vi "SEE_PXI_TopBench_Rev11.vi"() -> ()   [LabVIEW 2019]
uses:
  Controls/DataBlockControl.ctl
  Controls/RFBlockControl.ctl
  <instrlib>/niScope/Controls/niScope vertical coupling.ctl
  Controls/PlotColorArray.ctl
panel:
  out "OscilloscopeInfoArray":T2(array[cluster]) {"vertical coupling" items=["AC", "DC", "Ground"]}
  out "DCPowerInfoArray":T3(array[cluster])
  out "RFBlockInfoArray":T4[](array[typedef])
  out "error in":errorcluster
  out "VISAPowerInfoArray":T5(array[cluster])
  out "Run Parameters":T6
  in  "stop":bool
  out "Configuration Dashboard":bool[](array[boolean])
  in  "Data Collection Block":bool
  in  "Oscilloscope Block":bool
  in  "Power Block":bool
  in  "RF Block":bool
  in  "Data Block":bool
  in  "Reset":bool
  # "Instructions:\nProgress through the configuration dashboard, note the arrays to the right to confirm settings. Once everything is configured, you can begin data collection"
  # "IMPORTANT NOTES\n\nALL LEDs must be lit up before you can begin data collection. Even if you don't need an RF source or oscilloscope, you still just open up the system and then exit (you don't need to configure one.\n\nAfter data collection, you will have the option to reset the system or keep the configuration.\n\nOnly press \"stop\" if you are completely done with collecting data or if the program does not allow you to open another subvi\n\nIf you get a \"running an implicit call\" just restart the program"
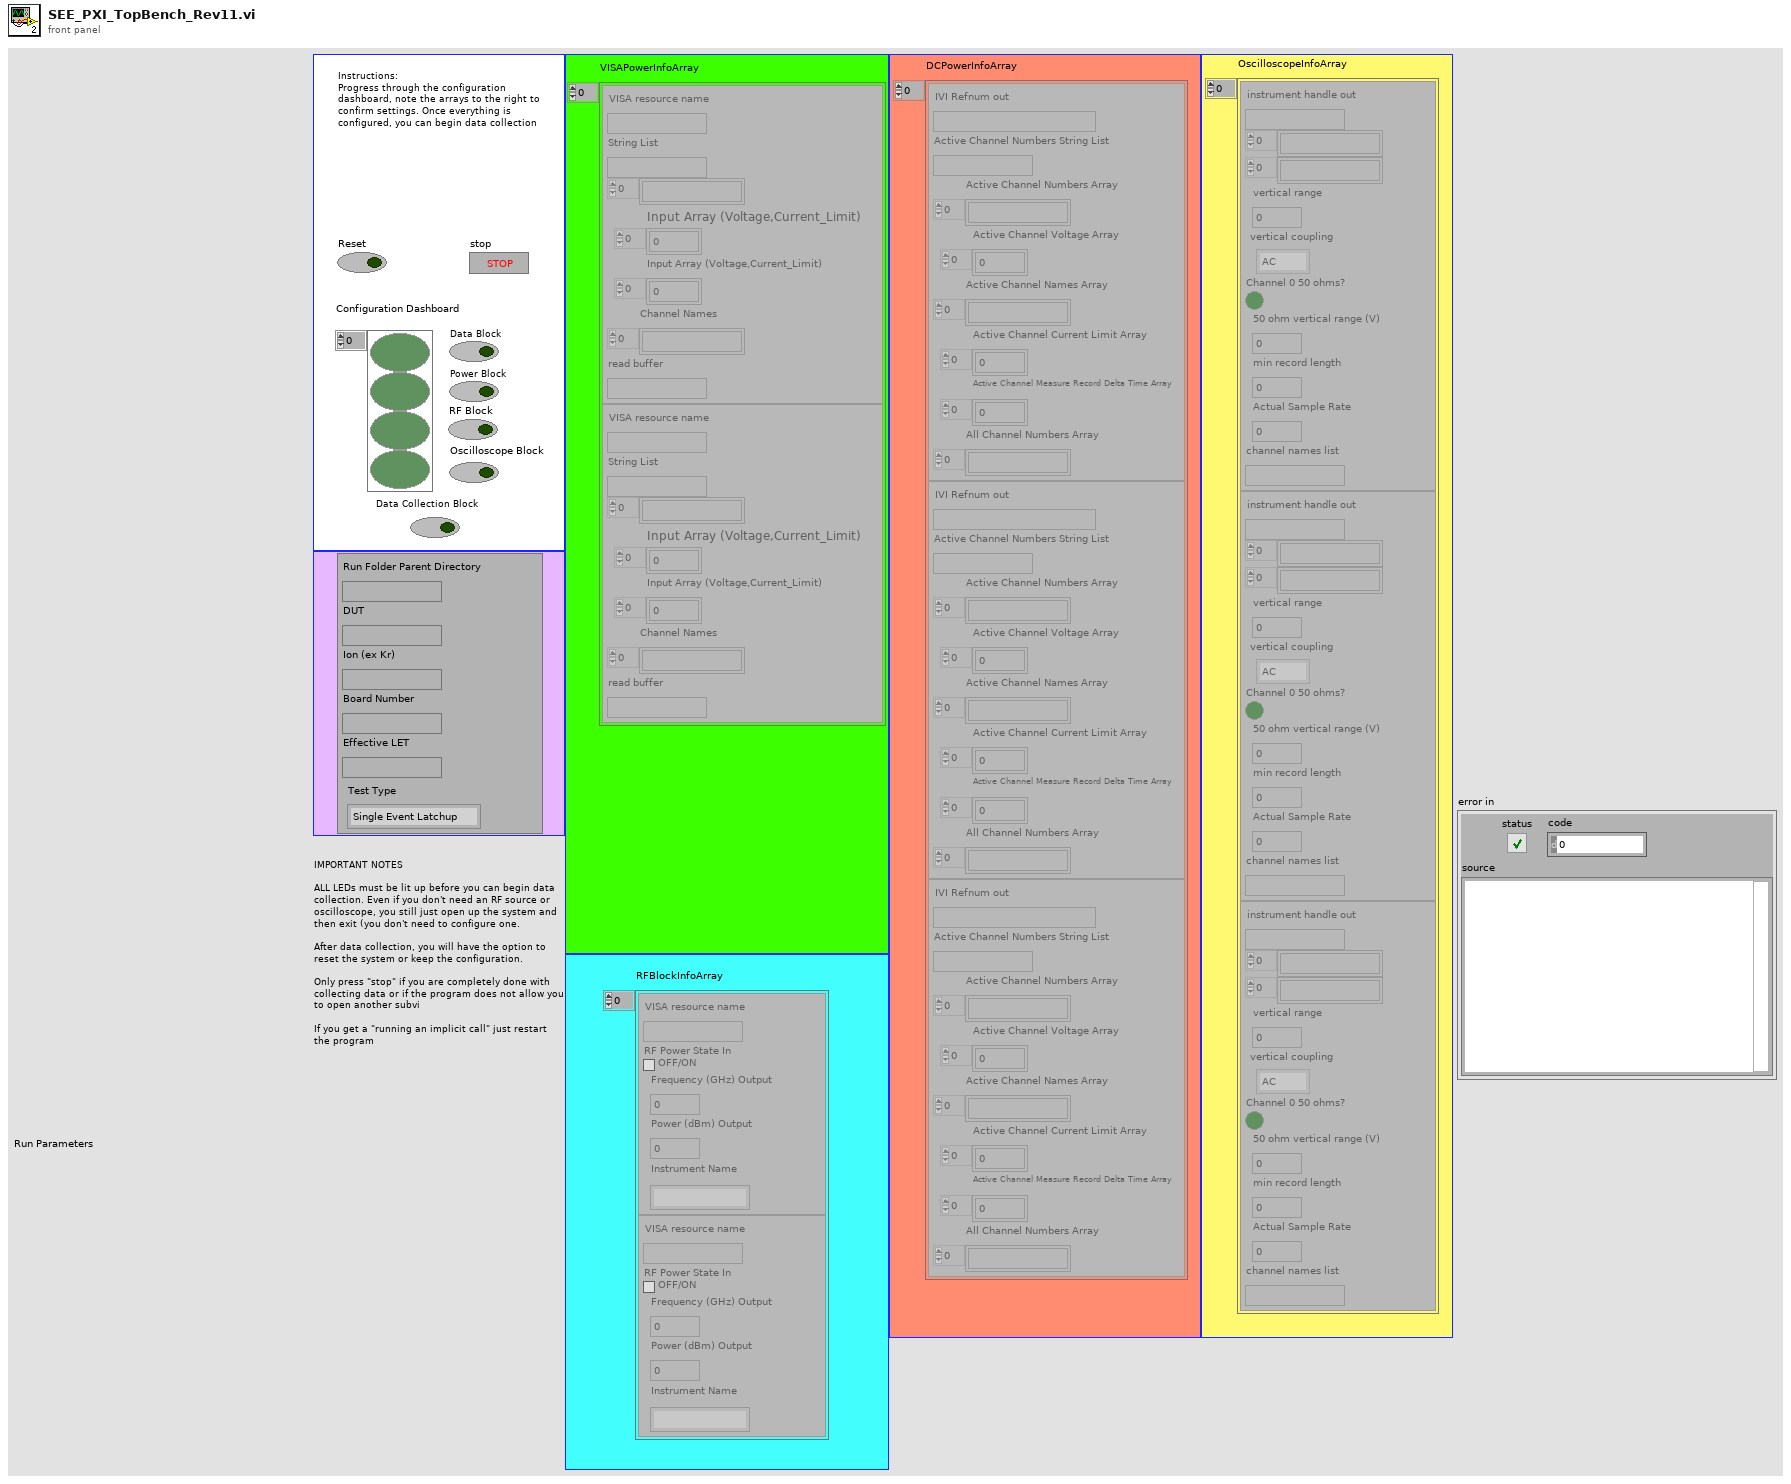
[diagram p1: front panel]
types:
  T1 = typedef "niScope vertical coupling.ctl" = i32
  T2 = cluster{"instrument handle out":refnum<k15>, string[], string[], "vertical range":dbl, "vertical coupling":T1, "Channel 0 50 ohms?":bool, "50 ohm vertical range (V)":dbl, "min record length":i32, "Actual Sample Rate":dbl, "channel names list":string}[]
  T3 = cluster{"IVI Refnum out":refnum<k15>, "Active Channel Numbers String List":string, "Active Channel Numbers Array":string[], "Active Channel Voltage Array":dbl[], "Active Channel Names Array":string[], "Active Channel Current Limit Array":dbl[], "Active Channel Measure Record Delta Time Array":dbl[], "All Channel Numbers Array":string[]}[]
  T4 = typedef "RFBlockControl.ctl" = cluster{"VISA resource name":refnum<visa-resource-name>, "RF Power State In":bool, "Frequency (GHz) Output":dbl, "Power (dBm) Output":dbl, "Instrument Name":string}
  T5 = cluster{"VISA resource name":refnum<visa-resource-name>, "String List":string, string[], "Input Array (Voltage,Current_Limit)":dbl[], "Input Array (Voltage,Current_Limit)":dbl[], "Channel Names":string[], "read buffer":string}[]
  T6 = typedef "DataBlockControl.ctl" = cluster{"Run Folder Parent Directory":path, "DUT":string, "Ion (ex Kr)":string, "Board Number":string, "Effective LET":string, "Test Type":enum16{"Single Event Latchup", "Single Event Transient", "Single Event Upset"}}
  T7 = typedef "PlotColorArray.ctl" = u32[]
  T8 = cluster{"instrument handle out":refnum<k15>, string, string[], dbl[], string[], "Current Limit Output Array":dbl[], dbl[]}[]
  T9 = cluster{"instrument handle out":refnum<k15>, "channel numbers array":string[], "channel names array":string[], "vertical range":dbl, "vertical coupling":T1, "Channel 0 50 ohms?":bool, "50 ohm vertical range (V)":dbl, "min record length":i32, "Actual Sample Rate":dbl}[]
  T10 = cluster{"Array of fetched data":dbl[][], string, i32[]}[]
  T11 = cluster{"Array of fetched data":dbl[][], string, i32[]}[][]
  T12 = cluster{"Array of fetched data":dbl[][], string, i32[]}
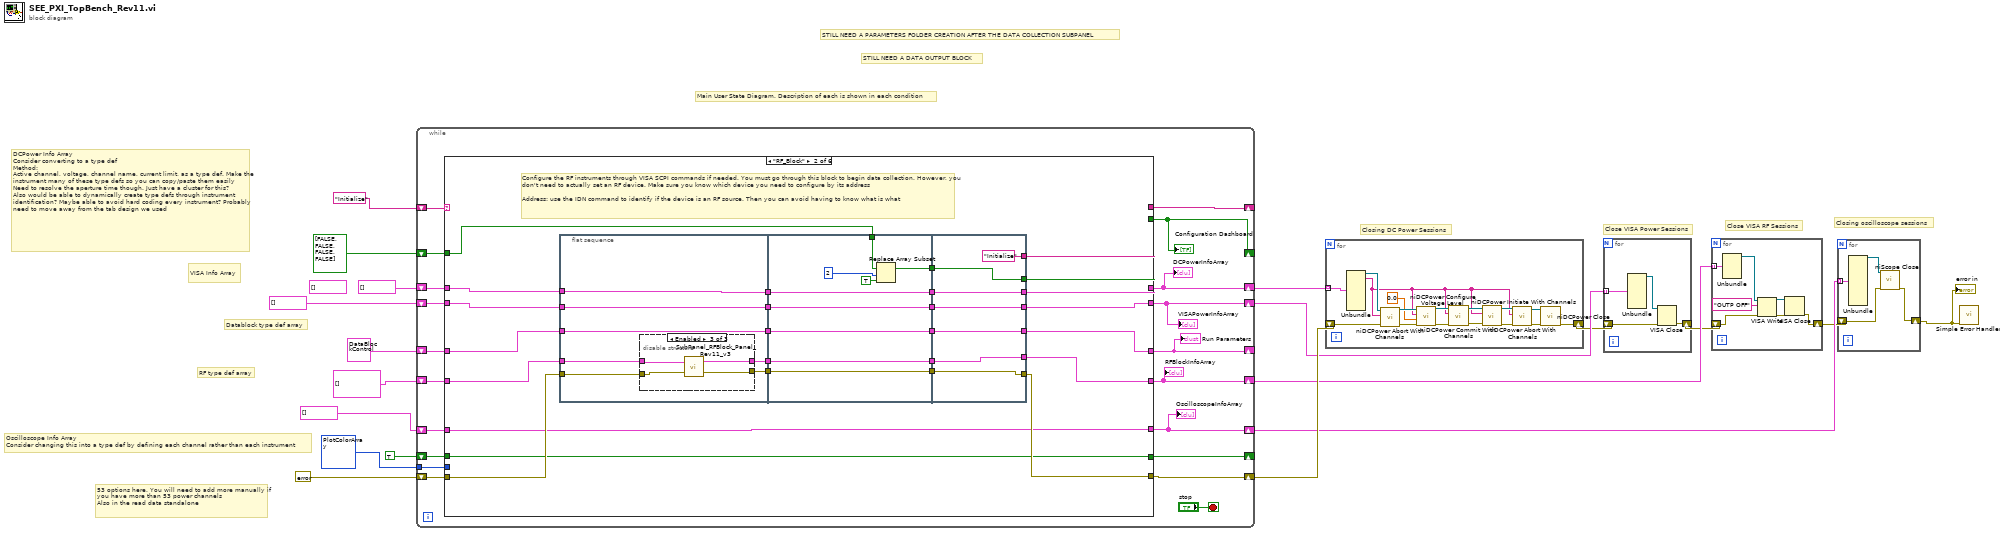
[diagram p0: block diagram]
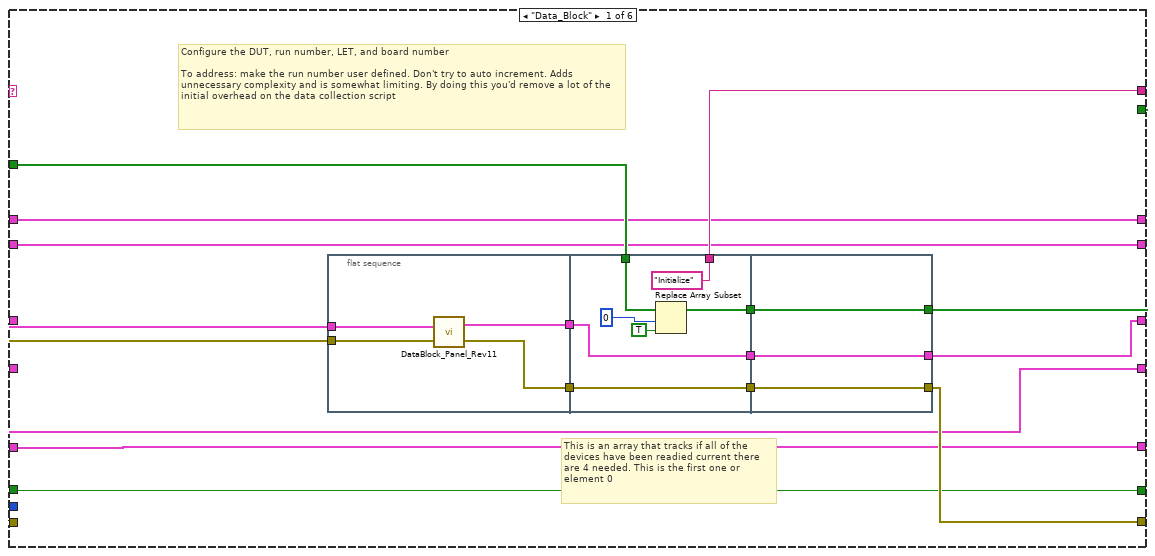
[diagram p2: hidden frame]
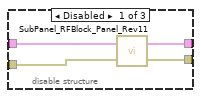
[diagram p3: hidden frame]
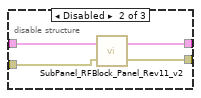
[diagram p4: hidden frame]
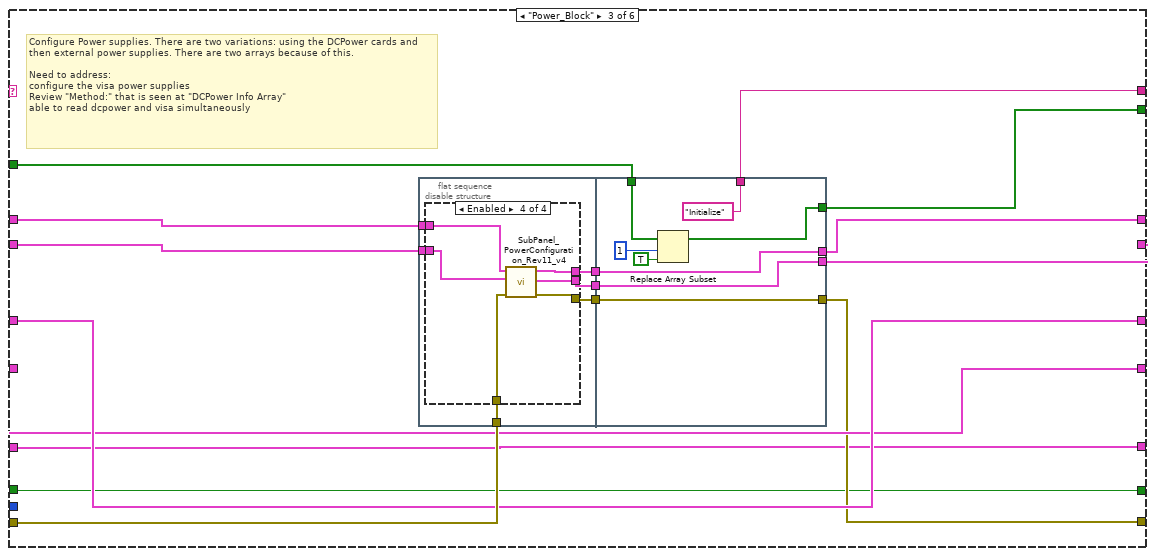
[diagram p5: hidden frame]
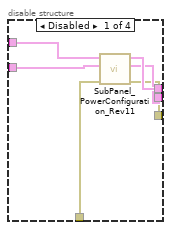
[diagram p6: hidden frame]
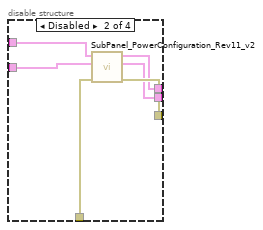
[diagram p7: hidden frame]
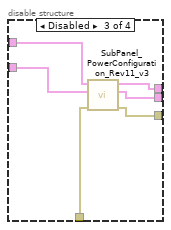
[diagram p8: hidden frame]
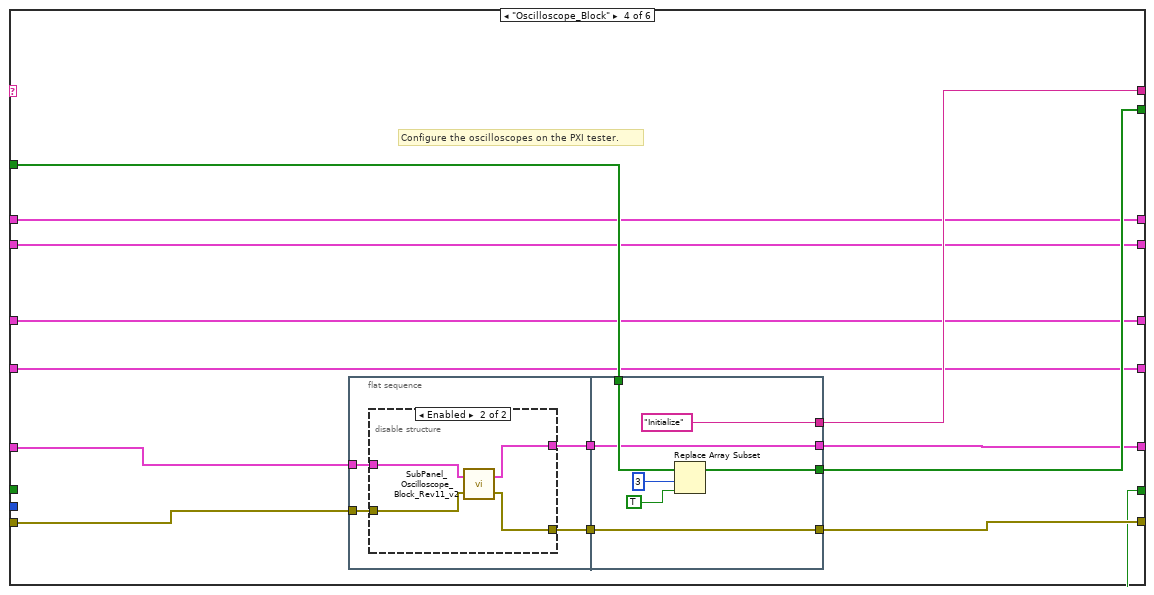
[diagram p9: hidden frame]
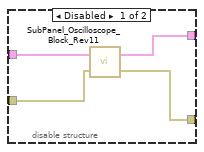
[diagram p10: hidden frame]
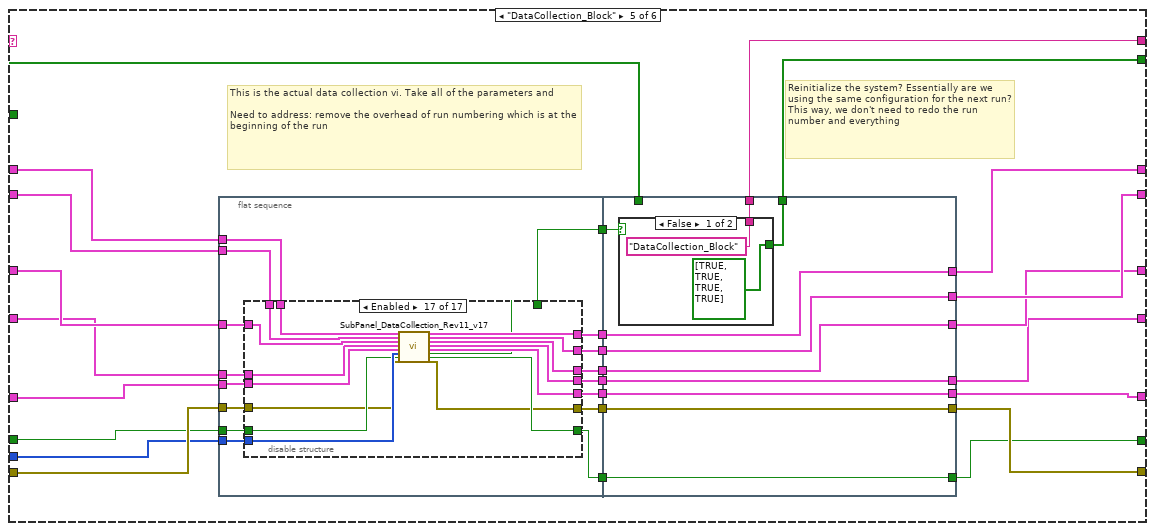
[diagram p11: hidden frame]
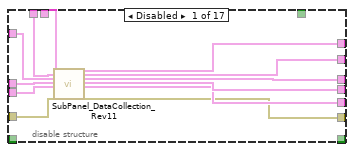
[diagram p12: hidden frame]
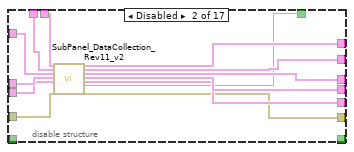
[diagram p13: hidden frame]
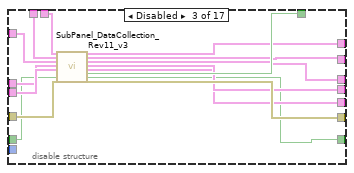
[diagram p14: hidden frame]
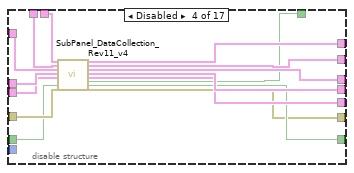
[diagram p15: hidden frame]
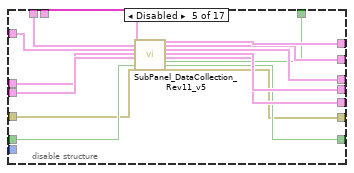
[diagram p16: hidden frame]
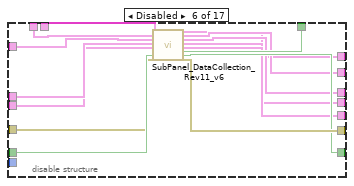
[diagram p17: hidden frame]
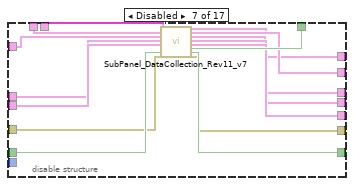
[diagram p18: hidden frame]
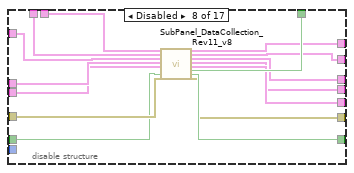
[diagram p19: hidden frame]
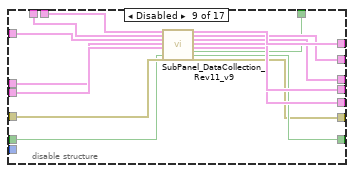
[diagram p20: hidden frame]
diagram:
  (unwired) T8 [] ("DCPowerInformationClusterArray_Input")
  # "Closing oscilloscope sessions"
  # "DCPower Info Array\nConsider converting to a type def\nMethod:\nActive channel, voltage, channel name, current limit, as a type def. Make the instrument many of these type defs so you can copy/paste them easily\nNeed to resolve the aperture time though. Just have a cluster for this?\nAlso would be able to dynamically create type defs through instrument identification? Maybe able to avoid hard coding every instrument? Probably need to move away from the tab design we used"
  # "Datablock type def array"
  # "RF type def array"
  # "Main User State Diagram. Description of each is shown in each condition"
  # "53 options here. You will need to add more manually if you have more than 53 power channels\nAlso in the read data standalone"
  # "STILL NEED A DATA OUTPUT BLOCK"
  # "STILL NEED A PARAMETERS FOLDER CREATION AFTER THE DATA COLLECTION SUBPANEL"
  # "Close VISA RF Sessions"
  # "Close VISA Power Sessions"
  # "Closing DC Power Sessions"
  # "Oscilloscope Info Array\nConsider changing this into a type def by defining each channel rather than each instrument"
  # "VISA Info Array"
  n1 = while {
    shift-right: [w37] -> _
    shift-left: bool[] [FALSE, FALSE, FALSE, FALSE] -> [w38]
    shift-right: [w36] -> _
    shift-left: "Initialize" -> [w39]
    shift-right: [w33] -> w13
    shift-left: errorcluster {"status"=FALSE, "code"=0, "source"=""} ("error in") -> [w34]
    shift-right: [w31] -> _
    shift-left: T6 {"Run Folder Parent Directory"=path "", "DUT"="", "Ion (ex Kr)"="", "Board Number"="", "Effective LET"="", "Test Type"=enum."Single Event Latchup"} ("Run Data SubPanel Input") -> [w32]
    shift-right: [w29] -> w10
    shift-left: T4[] [] ("RF Block Input Array") -> [w30]
    shift-right: [w25] -> w14
    shift-left: T3 [] ("DCPowerInformationClusterArray_Input") -> [w28]
    shift-right: [w26] -> w12
    shift-left: T5 [] ("VISAPowerInfoInputArray") -> [w27]
    shift-right: [w23] -> w6
    shift-left: T2 [] ("Oscilloscope Configuration Input Array") -> [w24]
    shift-right: [w21] -> _
    shift-left: TRUE ("New Run?") -> [w22]
    tunnel: T7 [16711686, 65351, 8978420, 14474240, 16139007, 16752640, 8958719, 16758973, 16777215, 46792, 11992992, 12961221, 16763690, 12600063, 16711835, 2953983, 40796, 13111296, 13352613, 9221011, 12964076, 12819897, 65442, 16776704, 14540253, 16740729, 10658047, 10813344, 16753521, 13413843, 8691115, 10339240, 14401205, 16746704, 7467519, 16775978, 13872558, 11387603, 13354405, 10420227, 13107364, 4060, 35208, 11817216, 7566080, 40796, 7539456, 2837073, 6372186, 7499083, 10648702, 16757152] ("Array") -> [w20]
    stop <- "stop" stop-if-true
    n2 = case shown="\"RF_Block\"" w39 {
      selector: w39 -> [_ _ _ _ _ w551]
      tunnel: w38 -> [w56 w93 w142 w199 w227 w553]
      tunnel: [w55 w92 w141 w198 w226 w552] -> w37
      tunnel: [w53 w96 w140 w197 w225 w549] -> w36
      tunnel: w34 -> [w52 w95 w145 w192 w239 w547]
      tunnel: [w51 w94 w134 w191 w229 w547] -> w33
      tunnel: w32 -> [w48 w82 w144 w194 w242 w546]
      tunnel: [w47 w81 w144 w194 w234 w546] -> w31
      tunnel: w30 -> [w44 w88 w143 w193 w241 w545]
      tunnel: [w44 w87 w143 w193 w232 w545] -> w29
      tunnel: w28 -> [w43 w77 w147 w196 w244 w544]
      tunnel: w27 -> [w42 w73 w146 w195 w243 w543]
      tunnel: [w43 w80 w139 w196 w238 w544] -> w25
      tunnel: [w42 w76 w137 w195 w236 w543] -> w26
      tunnel: w24 -> [w41 w72 w133 w189 w240 w542]
      tunnel: [w41 w72 w133 w188 w219 w542] -> w23
      tunnel: w22 -> [w40 w71 w132 w186 w223 w541]
      tunnel: [w40 w71 w132 w186 w221 w541] -> w21
      tunnel: w20 -> [_ _ _ _ w220 _]
      frame "Data_Block" {
        # "This is an array that tracks if all of the devices have been readied current there are 4 needed. This is the first one or element 0"
        # "Configure the DUT, run number, LET, and board number\n\nTo address: make the run number user defined. Don't try to auto increment. Adds unnecessary complexity and is somewhat limiting. By doing this you'd remove a lot of the initial overhead on the data collection script"
        n3 = flat-sequence {
          tunnel: w52 -> [w60]
          tunnel: [w59] -> w49
          tunnel: w48 -> [w58]
          tunnel: [w57] -> w45
          tunnel: w56 -> [w67]
          tunnel: [w64] -> w54
          tunnel: ["Initialize"] -> w53
          tunnel: [w62] -> w50
          tunnel: w49 -> [w62]
          tunnel: [w61] -> w46
          tunnel: w45 -> [w61]
          tunnel: [w70] -> w55
          tunnel: w54 -> [w70]
          tunnel: [w69] -> w51
          tunnel: w50 -> [w69]
          tunnel: [w68] -> w47
          tunnel: w46 -> [w68]
          frame #0 {
            n4 = call "DataBlock_Panel_Rev11.vi"("error in"=w60, "Run Data SubPanel Input"=w58) -> ("error out"=w59:errorcluster, "Run Data SubPanel Output"=w57:T6)
          }
          frame #1 {
            n5 = Replace Array Subset(array=w67, new element=TRUE ("new element/subarray"), index=0) -> (w64:bool[])
          }
          frame #2 {
          }
        }
      }
      frame "RF_Block" {
        # "Configure the RF instruments through VISA SCPI commands if needed. You must go through this block to begin data collection. However, you don't need to actually set an RF device. Make sure you know which device you need to configure by its address\n\nAddress: use the IDN command to identify if the device is an RF source. Then you can avoid having to know what is what"
        n6 = flat-sequence {
          tunnel: w95 -> [w103]
          tunnel: [w102] -> w89
          tunnel: w88 -> [w101]
          tunnel: [w100] -> w85
          tunnel: [w99] -> w83
          tunnel: w82 -> [w99]
          tunnel: [w98] -> w78
          tunnel: w77 -> [w98]
          tunnel: [w97] -> w74
          tunnel: w73 -> [w97]
          tunnel: w93 -> [w124]
          tunnel: [w121] -> w91
          tunnel: [w120] -> w90
          tunnel: w89 -> [w120]
          tunnel: [w119] -> w86
          tunnel: w85 -> [w119]
          tunnel: [w118] -> w84
          tunnel: w83 -> [w118]
          tunnel: [w117] -> w79
          tunnel: w78 -> [w117]
          tunnel: [w116] -> w75
          tunnel: w74 -> [w116]
          tunnel: ["Initialize"] -> w96
          tunnel: [w129] -> w94
          tunnel: [w130] -> w92
          tunnel: w91 -> [w130]
          tunnel: w90 -> [w129]
          tunnel: [w128] -> w87
          tunnel: w86 -> [w128]
          tunnel: [w127] -> w81
          tunnel: w84 -> [w127]
          tunnel: [w126] -> w80
          tunnel: w79 -> [w126]
          tunnel: [w125] -> w76
          tunnel: w75 -> [w125]
          frame #0 {
            n7 = disable-structure shown="Enabled" {
              disable-tunnel: w103 -> [w107 w110 w114]
              disable-tunnel: [w106 w108 w113] -> w102
              disable-tunnel: w101 -> [w105 w111 w115]
              disable-tunnel: [w104 w109 w112] -> w100
              frame Disabled {
                n8 = call "SubPanel_RFBlock_Panel_Rev11.vi"("error input"=w107, "RF Block Input"=w105) -> ("error output"=w106:errorcluster, "RF Block Output"=w104:T4)
              }
              frame Disabled {
                n9 = call "SubPanel_RFBlock_Panel_Rev11_v2.vi"("error input"=w110, "RF Block Input Array"=w111) -> ("error output"=w108:errorcluster, "RF Block Output Array"=w109:T4[])
              }
              frame Enabled {
                n10 = call "SubPanel_RFBlock_Panel_Rev11_v3.vi"("error input"=w114, "RF Block Input Array"=w115) -> ("error output"=w113:errorcluster, "RF Block Output Array"=w112:T4[])
              }
            }
          }
          frame #1 {
            n11 = Replace Array Subset(array=w124, new element=TRUE ("new element/subarray"), index=2) -> (w121:bool[])
          }
          frame #2 {
          }
        }
      }
      frame "Power_Block" {
        # "Configure Power supplies. There are two variations: using the DCPower cards and then external power supplies. There are two arrays because of this.  \n\nNeed to address:\nconfigure the visa power supplies\nReview \"Method:\" that is seen at \"DCPower Info Array\"\nable to read dcpower and visa simultaneously"
        n12 = flat-sequence {
          tunnel: w147 -> [w153]
          tunnel: w146 -> [w152]
          tunnel: w145 -> [w151]
          tunnel: [w150] -> w138
          tunnel: [w149] -> w136
          tunnel: [w148] -> w135
          tunnel: w142 -> [w183]
          tunnel: [w182] -> w141
          tunnel: ["Initialize"] -> w140
          tunnel: [w180] -> w139
          tunnel: w138 -> [w180]
          tunnel: [w179] -> w137
          tunnel: w136 -> [w179]
          tunnel: [w178] -> w134
          tunnel: w135 -> [w178]
          frame #0 {
            n13 = disable-structure shown="Enabled" {
              disable-tunnel: w153 -> [w159 w160 w168 w173]
              disable-tunnel: w152 -> [w158 w161 w167 w172]
              disable-tunnel: w151 -> [w157 w165 w166 w177]
              disable-tunnel: [w156 w162 w169 w174] -> w150
              disable-tunnel: [w155 w163 w170 w175] -> w149
              disable-tunnel: [w154 w164 w171 w176] -> w148
              frame Disabled {
                n14 = call "SubPanel_PowerConfiguration_Rev11.vi"("error in"=w157, "VISAPowerInfoInputArray"=w158, "DCPowerInformationClusterArray_Input"=w159) -> ("error out"=w154:errorcluster, "VISAPowerInfoOutputArray"=w155:T5, "DCPowerInformationClusterArray_Output"=w156:T8)  [unwired: 6 in]
              }
              frame Disabled {
                n15 = call "SubPanel_PowerConfiguration_Rev11_v2.vi"("error in"=w165, "VISAPowerInfoInputArray"=w161, "DCPowerInformationClusterArray_Input"=w160) -> ("error out"=w164:errorcluster, "VISAPowerInfoOutputArray"=w163:T5, "DCPowerInformationClusterArray_Output"=w162:T3)  [unwired: 6 in]
              }
              frame Disabled {
                n16 = call "SubPanel_PowerConfiguration_Rev11_v3.vi"("error in"=w166, "VISAPowerInfoInputArray"=w167, "DCPowerInformationClusterArray_Input"=w168) -> ("error out"=w171:errorcluster, "VISAPowerInfoOutputArray"=w170:T5, "DCPowerInformationClusterArray_Output"=w169:T3)  [unwired: 6 in]
              }
              frame Enabled {
                n17 = call "SubPanel_PowerConfiguration_Rev11_v4.vi"("error in"=w177, "VISAPowerInfoInputArray"=w172, "DCPowerInformationClusterArray_Input"=w173) -> ("error out"=w176:errorcluster, "VISAPowerInfoOutputArray"=w175:T5, "DCPowerInformationClusterArray_Output"=w174:T3)  [unwired: 6 in]
              }
            }
          }
          frame #1 {
            n18 = Replace Array Subset(array=w183, new element=TRUE ("new element/subarray"), index=1) -> (w182:bool[])
          }
        }
      }
      frame "Oscilloscope_Block" {
        # "Configure the oscilloscopes on the PXI tester."
        n19 = flat-sequence {
          tunnel: w192 -> [w203]
          tunnel: [w202] -> w190
          tunnel: w189 -> [w201]
          tunnel: [w200] -> w187
          tunnel: w199 -> [w218]
          tunnel: [w215] -> w198
          tunnel: ["Initialize"] -> w197
          tunnel: [w213] -> w191
          tunnel: w190 -> [w213]
          tunnel: [w212] -> w188
          tunnel: w187 -> [w212]
          frame #0 {
            n20 = disable-structure shown="Enabled" {
              disable-tunnel: w203 -> [w207 w209]
              disable-tunnel: [w206 w208] -> w202
              disable-tunnel: w201 -> [w205 w211]
              disable-tunnel: [w204 w210] -> w200
              frame Disabled {
                n21 = call "SubPanel_Oscilloscope_Block_Rev11.vi"("error input"=w207, "Oscilloscope Configuration Input Array"=w205) -> ("error out"=w206:errorcluster, "Oscilloscope Configuration Output Array"=w204:T9)
              }
              frame Enabled {
                n22 = call "SubPanel_Oscilloscope_Block_Rev11_v2.vi"("error input"=w209, "Oscilloscope Configuration Input Array"=w211) -> ("error out"=w208:errorcluster, "Oscilloscope Configuration Output Array"=w210:T2)
              }
            }
          }
          frame #1 {
            n23 = Replace Array Subset(array=w218, new element=TRUE ("new element/subarray"), index=3) -> (w215:bool[])
          }
        }
      }
      frame "DataCollection_Block" {
        # "Reinitialize the system? Essentially are we using the same configuration for the next run? This way, we don't need to redo the run number and everything"
        # "This is the actual data collection vi. Take all of the parameters and \n\nNeed to address: remove the overhead of run numbering which is at the beginning of the run"
        n24 = flat-sequence {
          tunnel: w244 -> [w260]
          tunnel: w243 -> [w259]
          tunnel: w242 -> [w258]
          tunnel: w241 -> [w257]
          tunnel: w240 -> [w256]
          tunnel: w239 -> [w255]
          tunnel: [w254] -> w237
          tunnel: [w253] -> w235
          tunnel: [w252] -> w233
          tunnel: [w251] -> w231
          tunnel: [w250] -> w230
          tunnel: [w249] -> w228
          tunnel: [w248] -> w224
          tunnel: w223 -> [w247]
          tunnel: [w246] -> w222
          tunnel: w220 -> [w245]
          tunnel: [w534] -> w238
          tunnel: w237 -> [w534]
          tunnel: [w533] -> w236
          tunnel: w235 -> [w533]
          tunnel: [w532] -> w234
          tunnel: w233 -> [w532]
          tunnel: [w531] -> w232
          tunnel: w231 -> [w531]
          tunnel: [w530] -> w219
          tunnel: w230 -> [w530]
          tunnel: [w529] -> w229
          tunnel: w228 -> [w529]
          tunnel: w227 -> [_]
          tunnel: [w528] -> w226
          tunnel: [w527] -> w225
          tunnel: w224 -> [w526]
          tunnel: [w525] -> w221
          tunnel: w222 -> [w525]
          frame #0 {
            n25 = disable-structure shown="Enabled" {
              disable-tunnel: w260 -> [w272 w278 w294 w320 w325 w354 w355 w376 w393 w414 w421 w444 w460 w468 w485 w508 w524]
              disable-tunnel: w259 -> [w271 w277 w295 w319 w326 w353 w356 w375 w394 w413 w420 w443 w459 w467 w484 w507 w523]
              disable-tunnel: w258 -> [w270 w276 w296 w310 w327 w352 w357 w374 w395 w412 w419 w442 w458 w466 w483 w506 w522]
              disable-tunnel: w257 -> [w269 w275 w297 w309 w328 w351 w358 w373 w396 w411 w418 w441 w457 w465 w482 w505 w521]
              disable-tunnel: w256 -> [w268 w274 w298 w308 w329 w350 w359 w372 w397 w410 w417 w440 w456 w464 w481 w504 w520]
              disable-tunnel: w255 -> [w267 w279 w300 w307 w330 w348 w360 w371 w399 w408 w415 w438 w455 w463 w478 w503 w517]
              disable-tunnel: [w266 w285 w292 w318 w339 w340 w362 w377 w392 w400 w422 w430 w446 w469 w486 w493 w516] -> w254
              disable-tunnel: [w265 w284 w291 w317 w338 w341 w363 w378 w391 w401 w423 w431 w447 w470 w487 w494 w515] -> w253
              disable-tunnel: [w264 w283 w290 w316 w337 w342 w364 w379 w390 w402 w424 w432 w448 w471 w488 w495 w514] -> w252
              disable-tunnel: [w263 w282 w289 w315 w336 w343 w365 w380 w389 w403 w425 w433 w449 w472 w489 w496 w513] -> w251
              disable-tunnel: [w262 w281 w288 w314 w335 w344 w366 w381 w388 w404 w426 w434 w450 w473 w477 w498 w512] -> w250
              disable-tunnel: [w261 w280 w299 w311 w332 w347 w367 w382 w385 w407 w427 w437 w451 w474 w490 w497 w509] -> w249
              disable-tunnel: [_ w273 w293 w313 w334 w345 w369 w384 w387 w405 w429 w435 w452 w476 w492 w499 w511] -> w248
              disable-tunnel: w247 -> [_ _ w287 w306 w331 w349 w361 w370 w398 w409 w416 w439 w454 w462 w479 w501 w518]
              disable-tunnel: [_ _ w286 w312 w333 w346 w368 w383 w386 w406 w428 w436 w453 w475 w491 w500 w510] -> w246
              disable-tunnel: w245 -> [_ _ _ _ _ _ _ _ _ _ _ _ w445 w461 w480 w502 w519]
              frame Disabled {
                n26 = call "SubPanel_DataCollection_Rev11.vi"("DCPowerInformationClusterArray_Input"=w272, "VISAPowerInfoInputArray"=w271, "Run Data SubPanel Input"=w270, "RF Block Parameters"=w269, "Oscilloscope Info Array"=w268, "error in"=w267) -> ("DCPowerInformationClusterArray_Output"=w266:T8, "VISAPowerInfoInputOutput"=w265:T5, "Run Data SubPanel Output"=w264:T6, "RF Block Parameters Output"=w263:T4, "Oscilloscope Info Array Output"=w262:T9, "error out"=w261:errorcluster)  [unwired: 16 in]
              }
              frame Disabled {
                n27 = call "SubPanel_DataCollection_Rev11_v2.vi"("DCPowerInformationClusterArray_Input"=w278, "VISAPowerInfoInputArray"=w277, "Run Data SubPanel Input"=w276, "RF Block Parameters"=w275, "Oscilloscope Info Array"=w274, "error in"=w279) -> ("DCPowerInformationClusterArray_Output"=w285:T8, "VISAPowerInfoInputOutput"=w284:T5, "Run Data SubPanel Output"=w283:T6, "RF Block Parameters Output"=w282:T4, "Oscilloscope Info Array Output"=w281:T9, "Reinitialize?"=w273:bool, "error out"=w280:errorcluster)  [unwired: 15 in]
              }
              frame Disabled {
                n28 = call "SubPanel_DataCollection_Rev11_v3.vi"("DCPowerInformationClusterArray_Input"=w294, "VISAPowerInfoInputArray"=w295, "Run Data SubPanel Input"=w296, "RF Block Parameters"=w297, "Oscilloscope Info Array"=w298, "New Run?"=w287, "error in"=w300) -> ("DCPowerInformationClusterArray_Output"=w292:T8, "VISAPowerInfoInputOutput"=w291:T5, "Run Data SubPanel Output"=w290:T6, "RF Block Parameters Output"=w289:T4, "Oscilloscope Info Array Output"=w288:T9, "Reinitialize?"=w293:bool, "Data Was Collected?"=w286:bool, "error out"=w299:errorcluster)  [unwired: 13 in]
              }
              frame Disabled {
                n29 = call "SubPanel_DataCollection_Rev11_v4.vi"("DCPowerInformationClusterArray_Input"=w320, "VISAPowerInfoInputArray"=w319, "Run Data SubPanel Input"=w310, "RF Block Parameters"=w309, "Oscilloscope Info Array"=w308, "New Run?"=w306, "error in"=w307) -> ("data iterating in loop"=w301:T10, "each channel cluster"=w302:T10, "Array of all channels?"=w305:dbl[][], "all channel clusters as a large array"=w303:T11, "data going into the binary file"=w304:T12, "DCPowerInformationClusterArray_Output"=w318:T8, "VISAPowerInfoInputOutput"=w317:T5, "Run Data SubPanel Output"=w316:T6, "RF Block Parameters Output"=w315:T4, "Oscilloscope Info Array Output"=w314:T9, "Reinitialize?"=w313:bool, "Data Was Collected?"=w312:bool, "error out"=w311:errorcluster)  [unwired: 8 in]
              }
              frame Disabled {
                n30 = call "SubPanel_DataCollection_Rev11_v5.vi"("DCPowerInformationClusterArray_Input"=w325, "VISAPowerInfoInputArray"=w326, "Run Data SubPanel Input"=w327, "RF Block Parameters"=w328, "Oscilloscope Info Array"=w329, "New Run?"=w331, "error in"=w330) -> ("data iterating in loop"=w322:T10, "each channel cluster"=w323:T10, "Array of all channels?"=w321:dbl[][], "all channel clusters as a large array"=w324:T11, "DCPowerInformationClusterArray_Output"=w339:T8, "VISAPowerInfoInputOutput"=w338:T5, "Run Data SubPanel Output"=w337:T6, "RF Block Parameters Output"=w336:T4, "Oscilloscope Info Array Output"=w335:T9, "Reinitialize?"=w334:bool, "Data Was Collected?"=w333:bool, "error out"=w332:errorcluster)  [unwired: 8 in, 1 out]
              }
              frame Disabled {
                n31 = call "SubPanel_DataCollection_Rev11_v6.vi"("DCPowerInformationClusterArray_Input"=w354, "VISAPowerInfoInputArray"=w353, "Run Data SubPanel Input"=w352, "RF Block Parameters"=w351, "Oscilloscope Info Array"=w350, "New Run?"=w349, "error in"=w348) -> ("DCPowerInformationClusterArray_Output"=w340:T8, "VISAPowerInfoInputOutput"=w341:T5, "Run Data SubPanel Output"=w342:T6, "RF Block Parameters Output"=w343:T4, "Oscilloscope Info Array Output"=w344:T9, "Reinitialize?"=w345:bool, "Data Was Collected?"=w346:bool, "error out"=w347:errorcluster)  [unwired: 13 in]
              }
              frame Disabled {
                n32 = call "SubPanel_DataCollection_Rev11_v7.vi"("DCPowerInformationClusterArray_Input"=w355, "VISAPowerInfoInputArray"=w356, "Run Data SubPanel Input"=w357, "RF Block Parameters"=w358, "Oscilloscope Info Array"=w359, "New Run?"=w361, "error in"=w360) -> ("DCPowerInformationClusterArray_Output"=w362:T8, "VISAPowerInfoInputOutput"=w363:T5, "Run Data SubPanel Output"=w364:T6, "RF Block Parameters Output"=w365:T4, "Oscilloscope Info Array Output"=w366:T9, "Reinitialize?"=w369:bool, "Data Was Collected?"=w368:bool, "error out"=w367:errorcluster)  [unwired: 12 in, 1 out]
              }
              frame Disabled {
                n33 = call "SubPanel_DataCollection_Rev11_v8.vi"("DCPowerInformationClusterArray_Input"=w376, "VISAPowerInfoInputArray"=w375, "Run Data SubPanel Input"=w374, "RF Block Parameters"=w373, "Oscilloscope Info Array"=w372, "New Run?"=w370, "error in"=w371) -> ("DCPowerInformationClusterArray_Output"=w377:T8, "VISAPowerInfoInputOutput"=w378:T5, "Run Data SubPanel Output"=w379:T6, "RF Block Parameters Output"=w380:T4, "Oscilloscope Info Array Output"=w381:T9, "Reinitialize?"=w384:bool, "Data Was Collected?"=w383:bool, "error out"=w382:errorcluster)  [unwired: 12 in, 1 out]
              }
              frame Disabled {
                n34 = call "SubPanel_DataCollection_Rev11_v9.vi"("DCPowerInformationClusterArray_Input"=w393, "VISAPowerInfoInputArray"=w394, "Run Data SubPanel Input"=w395, "RF Block Parameters"=w396, "Oscilloscope Info Array"=w397, "New Run?"=w398, "error in"=w399) -> ("DCPowerInformationClusterArray_Output"=w392:T8, "VISAPowerInfoInputOutput"=w391:T5, "Run Data SubPanel Output"=w390:T6, "RF Block Parameters Output"=w389:T4, "Oscilloscope Info Array Output"=w388:T9, "Reinitialize?"=w387:bool, "Data Was Collected?"=w386:bool, "error out"=w385:errorcluster)  [unwired: 13 in]
              }
              frame Disabled {
                n35 = call "SubPanel_DataCollection_Rev11_v10.vi"("DCPowerInformationClusterArray_Input"=w414, "VISAPowerInfoInputArray"=w413, "Run Data SubPanel Input"=w412, "RF Block Parameters"=w411, "Oscilloscope Info Array"=w410, "New Run?"=w409, "error in"=w408) -> ("DCPowerInformationClusterArray_Output"=w400:T8, "VISAPowerInfoInputOutput"=w401:T5, "Run Data SubPanel Output"=w402:T6, "RF Block Parameters Output"=w403:T4, "Oscilloscope Info Array Output"=w404:T9, "Reinitialize?"=w405:bool, "Data Was Collected?"=w406:bool, "error out"=w407:errorcluster)  [unwired: 13 in]
              }
              frame Disabled {
                n36 = call "SubPanel_DataCollection_Rev11_v11.vi"("DCPowerInformationClusterArray_Input"=w421, "VISAPowerInfoInputArray"=w420, "Run Data SubPanel Input"=w419, 3:w418, "Oscilloscope Info Array"=w417, "New Run?"=w416, "error in"=w415) -> ("DCPowerInformationClusterArray_Output"=w422:T8, "VISAPowerInfoInputOutput"=w423:T5, "Run Data SubPanel Output"=w424:T6, "RF Block Parameters Output"=w425:T4, "Oscilloscope Info Array Output"=w426:T9, "Reinitialize?"=w429:bool, "Data Was Collected?"=w428:bool, "error out"=w427:errorcluster)  [unwired: 13 in]
              }
              frame Disabled {
                n37 = call "SubPanel_DataCollection_Rev11_v12.vi"("DCPowerInformationClusterArray_Input"=w444, "VISAPowerInfoInputArray"=w443, "Run Data SubPanel Input"=w442, "RF Block Input Array"=w441, "Oscilloscope Info Array"=w440, "New Run?"=w439, "error in"=w438) -> ("DCPowerInformationClusterArray_Output"=w430:T8, "VISAPowerInfoInputOutput"=w431:T5, "Run Data SubPanel Output"=w432:T6, "RF Subpanel Output"=w433:T4[], "Oscilloscope Info Array Output"=w434:T9, "Reinitialize?"=w435:bool, "Data Was Collected?"=w436:bool, "error out"=w437:errorcluster)  [unwired: 13 in]
              }
              frame Disabled {
                n38 = call "SubPanel_DataCollection_Rev11_v13.vi"("DCPowerInformationClusterArray_Input"=w460, "VISAPowerInfoInputArray"=w459, "Run Data SubPanel Input"=w458, "RF Block Input Array"=w457, "Oscilloscope Info Array"=w456, "Plot Color Array"=w445, "New Run?"=w454, "error in"=w455) -> ("DCPowerInformationClusterArray_Output"=w446:T8, "VISAPowerInfoInputOutput"=w447:T5, "Run Data SubPanel Output"=w448:T6, "RF Subpanel Output"=w449:T4[], "Oscilloscope Info Array Output"=w450:T9, "Reinitialize?"=w452:bool, "Data Was Collected?"=w453:bool, "error out"=w451:errorcluster)  [unwired: 12 in]
              }
              frame Disabled {
                n39 = call "SubPanel_DataCollection_Rev11_v14.vi"("DCPowerInformationClusterArray_Input"=w468, "VISAPowerInfoInputArray"=w467, "Run Data SubPanel Input"=w466, "RF Block Input Array"=w465, "Oscilloscope Info Array"=w464, "Plot Color Array"=w461, "New Run?"=w462, "error in"=w463) -> ("DCPowerInformationClusterArray_Output"=w469:T8, "VISAPowerInfoInputOutput"=w470:T5, "Run Data SubPanel Output"=w471:T6, "RF Subpanel Output"=w472:T4[], "Oscilloscope Info Array Output"=w473:T9, "Reinitialize?"=w476:bool, "Data Was Collected?"=w475:bool, "error out"=w474:errorcluster)  [unwired: 12 in]
              }
              frame Disabled {
                n40 = call "SubPanel_DataCollection_Rev11_v15.vi"("DCPowerInformationClusterArray_Input"=w485, "VISAPowerInfoInputArray"=w484, "Run Data SubPanel Input"=w483, "RF Block Input Array"=w482, "Oscilloscope Info Array"=w481, "Plot Color Array"=w480, "New Run?"=w479, "error in"=w478) -> ("DCPowerInformationClusterArray_Output"=w486:T8, "VISAPowerInfoInputOutput"=w487:T5, "Run Data SubPanel Output"=w488:T6, "RF Subpanel Output"=w489:T4[], "Oscilloscope Info Array"=w477:T2, "Reinitialize?"=w492:bool, "Data Was Collected?"=w491:bool, "error out"=w490:errorcluster)  [unwired: 12 in]
              }
              frame Disabled {
                n41 = call "SubPanel_DataCollection_Rev11_v16.vi"("DCPowerInformationClusterArray_Input"=w508, "VISAPowerInfoInputArray"=w507, "Run Data SubPanel Input"=w506, "RF Block Input Array"=w505, "Oscilloscope Info Array"=w504, "Plot Color Array"=w502, "New Run?"=w501, "error in"=w503) -> ("DCPowerInformationClusterArray_Output"=w493:T3, "VISAPowerInfoInputOutput"=w494:T5, "Run Data SubPanel Output"=w495:T6, "RF Subpanel Output"=w496:T4[], "Oscilloscope Info Array"=w498:T2, "Reinitialize?"=w499:bool, "Data Was Collected?"=w500:bool, "error out"=w497:errorcluster)  [unwired: 12 in]
              }
              frame Enabled {
                n42 = call "SubPanel_DataCollection_Rev11_v17.vi"("DCPowerInformationClusterArray_Input"=w524, "VISAPowerInfoInputArray"=w523, "Run Data SubPanel Input"=w522, "RF Block Input Array"=w521, "Oscilloscope Info Array"=w520, "Plot Color Array"=w519, "New Run?"=w518, "error in"=w517) -> ("DCPowerInformationClusterArray_Output"=w516:T3, "VISAPowerInfoInputOutput"=w515:T5, "Run Data SubPanel Output"=w514:T6, "RF Subpanel Output"=w513:T4[], "Oscilloscope Info Array"=w512:T2, "Reinitialize?"=w511:bool, "Data Was Collected?"=w510:bool, "error out"=w509:errorcluster)  [unwired: 12 in]
              }
            }
          }
          frame #1 {
            n43 = case shown="False" w526 {
              tunnel: [bool[] [TRUE, TRUE, TRUE, TRUE] bool[] [FALSE, FALSE, FALSE, FALSE]] -> w528
              tunnel: ["DataCollection_Block" "Initialize"] -> w527
              frame False {
              }
              frame True {
              }
            }
          }
        }
      }
      frame "Initialize", Default {
        # "Forces you to always set up where you want to put the data first"
        # "This checks if you have completed all of the instrument configuration pages. You will not be able to begin data collection if you don't"
        # "The \"standby\" or \"idle\" loop. You control which configuration panel you're going into from here"
        n44 = case shown="True" "Reset" {
          tunnel: w553 -> [w614 _]
          tunnel: [w614 bool[] [FALSE, FALSE, FALSE, FALSE]] -> w552
          tunnel: [w612 w615] -> w560
          tunnel: w551 -> [w612 w615]
          frame False {
            n45 = Wait (ms)(milliseconds to wait=u32 50) -> ()  [unwired: 1 out]
          }
          frame True {
          }
        }
        n46 = Build Array("Data Block", "Power Block", "RF Block", "Oscilloscope Block", "Data Collection Block") -> (w559:bool[])
        n47 = for {
          tunnel: w559 -> [w608] mode=indexing
          shift-right: [w607] -> w548
          shift-left: 0 -> [w606]
          tunnel: [w604] -> w550
          tunnel: w560 -> [w604]
          i -> [w609]
          n48 = Increment(x=w609) -> (x+1=w605:i32)
          n49 = case shown="True" w608 {
            tunnel: [w610 w611] -> w607
            tunnel: w606 -> [w610 _]
            tunnel: w605 -> [_ w611]
            frame False {
            }
            frame True {
            }
          }
        }
        n50 = case shown="3" w548 {
          tunnel: [w561 "Data_Block" w567 w574 w584 w592] -> w549
          tunnel: w550 -> [w561 _ _ _ _ _]
          tunnel: w552 -> [_ _ w564 w571 w583 w590]
          frame 0, Default {
            n51 = flat-sequence {
              frame #0 {
                n52 = Wait (ms)(milliseconds to wait=u32 50) -> ()  [unwired: 1 out]
              }
              frame #1 {
              }
            }
          }
          frame 1 {
          }
          frame 3 {
            n53 = Index Array(array=w564, index=0) -> (element=w565:bool)
            n54 = case shown="False" w565 {
              tunnel: ["Data_Block" "RF_Block"] -> w567
              frame False {
                n55 = call "Display Message to User"("Message"="Please Configure the DUT information before continuing") -> ()  [unwired: 9 in, 2 out]
              }
              frame True {
              }
            }
          }
          frame 2 {
            n56 = Index Array(array=w571, index=0) -> (element=w572:bool)
            n57 = case shown="False" w572 {
              tunnel: [w575 "Power_Block"] -> w574
              frame False {
                n58 = Two Button Dialog(message="Please Configure the DUT information before continuing", 1:"Ok" ("F button name (\"Cancel\")"), 2:"I'm going in anyway" ("T button name (\"OK\")")) -> (T button?=w576:bool)
                n59 = case shown="True" w576 {
                  tunnel: ["Data_Block" "Power_Block"] -> w575
                  frame False {
                  }
                  frame True {
                  }
                }
              }
              frame True {
              }
            }
          }
          frame 4 {
            n60 = Index Array(array=w583, index=0) -> (element=w585:bool)
            n61 = case shown="False" w585 {
              tunnel: ["Data_Block" "Oscilloscope_Block"] -> w584
              frame False {
                n62 = call "Display Message to User3"("Message"="Please Configure the DUT information before continuing") -> ()  [unwired: 9 in, 2 out]
              }
              frame True {
              }
            }
          }
          frame 5 {
            n63 = disable-structure shown="Disabled" {
              disable-tunnel: [w594 w599] -> w591
              disable-tunnel: w590 -> [w593 w600]
              frame Disabled {
                n64 = for {
                  tunnel: w593 -> [w598] mode=indexing
                  shift-right: [w596] -> w594
                  shift-left: TRUE ("y") -> [w597]
                  n65 = And(x=w598, y=w597) -> (x .and. y?=w596:bool)
                }
              }
              frame Enabled {
                n66 = And Array Elements(Boolean array=w600) -> (logical AND=w599:bool)
              }
            }
            n67 = case shown="False" w591 {
              tunnel: ["Initialize" "DataCollection_Block"] -> w592
              frame False {
                n68 = call "Display Message to User4"("Message"="Ensure you have configured everything") -> ()  [unwired: 9 in, 2 out]
              }
              frame True {
              }
            }
          }
        }
      }
    }
    "Configuration Dashboard" <- w37
    "Run Parameters" <- w31
    "VISAPowerInfoArray" <- w26
    "RFBlockInfoArray" <- w29
    "DCPowerInfoArray" <- w25
    "OscilloscopeInfoArray" <- w23
  }
  n69 = for {
    tunnel: w14 -> [w632] mode=indexing
    shift-right: [w631] -> w11
    shift-left: w13 -> [w627]
    n70 = Unbundle(w632) -> ("IVI Refnum out"=w628:refnum<k15>, "Active Channel Numbers String List"=w617:string)  [unwired: 6 out]
    n71 = call <instrlib>:"niDCPower Abort With Channels.vi"("error in (no error)"=w627, "channel name"=w617, "instrument handle"=w628) -> ("error out"=w630:errorcluster, "instrument handle out"=w629:refnum<k15>)  [unwired: 7 in]
    n72 = call <instrlib>:"niDCPower Configure Voltage Level.vi"("error in (no error)"=w630, "voltage level"=0.0, "channel name"=w617, "instrument handle"=w629) -> ("error out"=w622:errorcluster, "instrument handle out"=w623:refnum<k15>)  [unwired: 6 in]
    n73 = call <instrlib>:"niDCPower Commit With Channels.vi"("error in (no error)"=w622, "channel name"=w617, "instrument handle"=w623) -> ("error out"=w624:errorcluster, "instrument handle out"=w625:refnum<k15>)  [unwired: 7 in]
    n74 = call <instrlib>:"niDCPower Initiate With Channels.vi"("error in (no error)"=w624, "channel name"=w617, "instrument handle"=w625) -> ("error out"=w619:errorcluster, "instrument handle out"=w618:refnum<k15>)  [unwired: 7 in]
    n75 = call <instrlib>:"niDCPower Abort With Channels.vi"("error in (no error)"=w619, "channel name"=w617, "instrument handle"=w618) -> ("error out"=w621:errorcluster, "instrument handle out"=w620:refnum<k15>)  [unwired: 7 in]
    n76 = call <instrlib>:"niDCPower Close.vi"("error in (no error)"=w621, "instrument handle"=w620) -> ("error out"=w631:errorcluster)  [unwired: 9 in]
  }
  n77 = for {
    tunnel: w12 -> [w636] mode=indexing
    shift-right: [w633] -> w9
    shift-left: w11 -> [w634]
    n78 = Unbundle(w636) -> ("VISA resource name"=w635:refnum<visa-resource-name>)  [unwired: 6 out]
    n79 = VISA Close(VISA resource name=w635, error in (no error)=w634) -> (error out=w633:errorcluster)
  }
  n80 = for {
    tunnel: w10 -> [w643] mode=indexing
    shift-right: [w642] -> w5
    shift-left: w9 -> [w639]
    n81 = Unbundle(w643) -> ("VISA resource name"=w638:refnum<visa-resource-name>)  [unwired: 4 out]
    n82 = VISA Write(VISA resource name=w638, write buffer="OUTP OFF", error in (no error)=w639) -> (VISA resource name out=w640:refnum<visa-resource-name>, error out=w641:errorcluster)  [unwired: 1 out]
    n83 = VISA Close(VISA resource name=w640, error in (no error)=w641) -> (error out=w642:errorcluster)
  }
  n84 = for {
    tunnel: w6 -> [w647] mode=indexing
    shift-right: [w645] -> w4
    shift-left: w5 -> [w646]
    n85 = Unbundle(w647) -> ("instrument handle out"=w644:refnum<k15>)  [unwired: 9 out]
    n86 = call <instrlib>:"niScope Close.vi"("instrument handle"=w644, "error in"=w646) -> ("error out"=w645:errorcluster)  [unwired: 13 in]
  }
  "error in" <- w4
  n87 = call <vilib>:"Simple Error Handler.vi"("error in (no error)"=w4) -> ()  [unwired: 4 in, 5 out]
